vi "ENCODER.vi"() -> ()   [LabVIEW 2017]
panel:
  in  "Reset_Z":bool
  out "Position_Z":i16
  in  "Reset_Y":bool
  out "Position_Y":i16
  out "Position_X":i16
  in  "Reset_X":bool
  in  "stop":bool
  # "Encoder Read X Y Z"
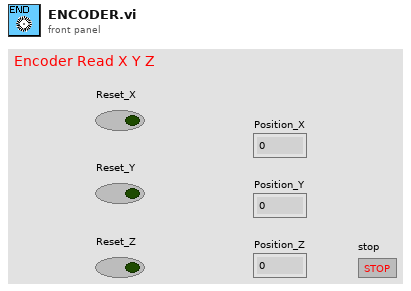
[diagram p1: front panel]
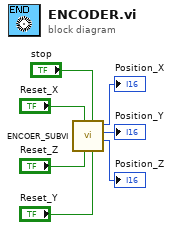
[diagram p0: block diagram]
diagram:
  n1 = call "ENCOER_SUBVI.vi"("Reset_Y"="Reset_Y", "stop"="stop", "Reset_Z"="Reset_Z", "Reset_X"="Reset_X") -> ("Position_Z"=→"Position_Z":i16, "Position_Y"=→"Position_Y":i16, "Position_X"=→"Position_X":i16)  [unwired: 5 in]
